vi "I2C Burst Write.vi"(9 "data":string, 10 "nBytes":i32, 11 "i2cAddress":u8) -> (1 "data out":string, 3 "function return":u32)   [LabVIEW 2018, in "AndorSDK.lvlib"]
doc: "EXPNETTYPE unsigned int WINAPI I2CBurstWrite(BYTE i2cAddress, long nBytes, BYTE * data);"
uses:
  AndorSDK.lvlib
  ATMCD32D.dll
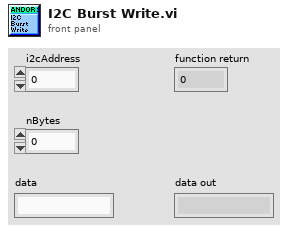
[diagram p1: front panel]
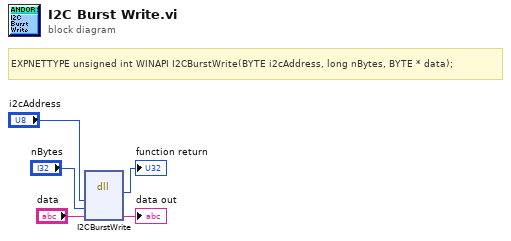
[diagram p0: block diagram]
diagram:
  # "EXPNETTYPE unsigned int WINAPI I2CBurstWrite(BYTE i2cAddress, long nBytes, BYTE * data);"
  n1 = dll-call lib="PTH2babs E\nPersönliches02 - Arbeit03-HiwijobsLabviewCodelibANDOR\tAndor SDK\nATMCD32D.*" fn="I2CBurstWrite"("i2cAddress"="i2cAddress", "nBytes"="nBytes", "data"="data") -> (→"function return":u32, "data"=→"data out":string)  [unwired: 5 in, 2 out]
